vi "WSVCAP SHL Host TL I2C Read.vi"(0 "Bytes to Read":u8=8, 5 "Sub Address [U8]":u8=191 format="%.0x", 7 "Socket Mask Set [U64]":u64[](array[numeric]) format="%012x", 11 "error in":errorcluster, 13 "Log (T)":bool=TRUE) -> (4 "C1 Read Data Out":u8[][](array[numeric]) format="%.0x", 6 "C2 Read Data Out":u8[][](array[numeric]) format="%.0x", 8 "C3 Read Data Out":u8[][](array[numeric]) format="%.0x", 15 "error out":errorcluster)   [LabVIEW 2012]
uses:
  Type Defs/WSVCAP SHL Function Enum.ctl
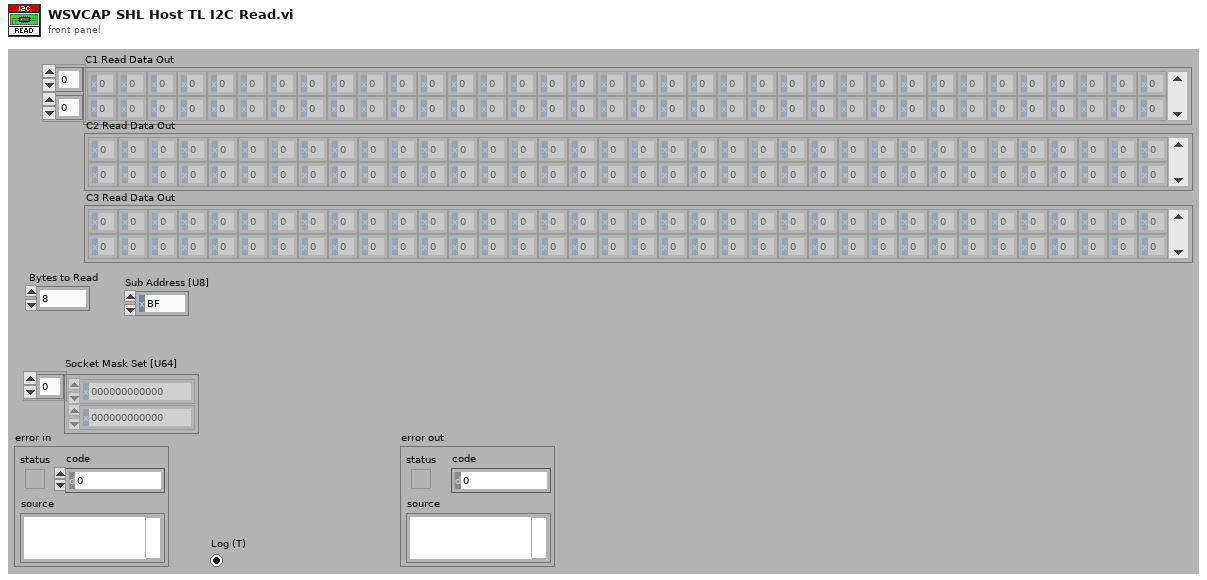
[diagram p1: front panel]
types:
  T1 = typedef "WSVCAP SHL Function Enum.ctl" = enum16{"Initialize", "Configure I2C", "Configure SPI", "Configure RFFE", "Write I2C", "Read I2C", "Write/Read SPI", "Start SPI Cycle", "Stop SPI Cycle", "Write RFFE", "Read RFFE", "Start RFFE Cycle", "Stop RFFE Cycle", "Get Status", "Close"}
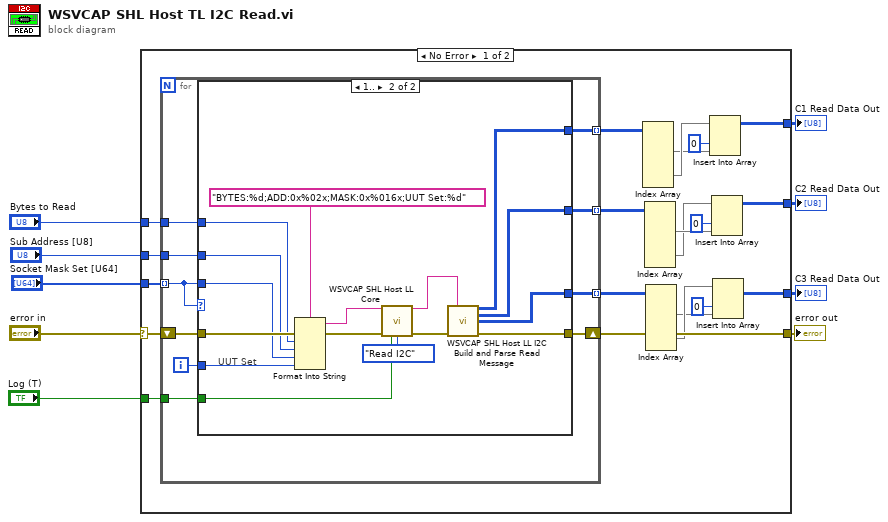
[diagram p0: block diagram]
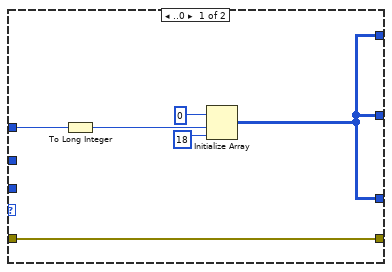
[diagram p2: hidden frame]
diagram:
  n1 = case shown="No Error" "error in" {
    selector: "error in" -> [w29 w63]
    tunnel: [w30 w63] -> w8
    tunnel: [w21 _] -> w3
    tunnel: [w12 _] -> w2
    tunnel: "Bytes to Read" -> [w28 _]
    tunnel: "Sub Address [U8]" -> [w27 _]
    tunnel: "Socket Mask Set [U64]" -> [w26 _]
    tunnel: "Log (T)" -> [w25 _]
    tunnel: [w10 _] -> w1
    frame No Error {
      n2 = for {
        tunnel: [w39] -> w13 mode=indexing
        tunnel: w28 -> [w37]
        tunnel: w27 -> [w36]
        tunnel: w26 -> [w33] mode=indexing
        tunnel: w25 -> [w35]
        tunnel: [w34] -> w11 mode=indexing
        tunnel: [w32] -> w20 mode=indexing
        shift-right: [w40] -> w30
        shift-left: w29 -> [w38]
        i -> [w31]
        n3 = case shown="1.." w33 {
          tunnel: [w46 w61] -> w40
          tunnel: [w42 w59] -> w32
          tunnel: [w42 w58] -> w39
          tunnel: w38 -> [w46 w57]
          tunnel: w37 -> [w43 w54]
          tunnel: w36 -> [_ w53]
          tunnel: w33 -> [_ w52]
          tunnel: w35 -> [_ w49]
          tunnel: [w42 w48] -> w34
          tunnel: w31 -> [_ w47]
          frame ..0 {
            n4 = To Long Integer(number=w43) -> (32bit integer=w41:i32)
            n5 = Initialize Array(u8 0 ("Read Data"), w41, 18 ("Read Data")) -> (w42:u8[][])
          }
          frame 1.. {
            # "UUT Set"
            n6 = Format Into String(format string="BYTES:%d;ADD:0x%02x;MASK:0x%016x;UUT Set:%d", error in=w57, w54, w53, w52, w47) -> (resulting string=w51:string, error out=w56:errorcluster)  [unwired: 1 in]
            n7 = call "WSVCAP SHL Host LL Core.vi"("Message In"=w51, "error in"=w56, "Log (T)"=w49, "Function"=WSVCAP_SHL_Function_Enum."Read I2C") -> ("Message Out"=w60:string, "error out"=w62:errorcluster)  [unwired: 9 in, 1 out]
            n8 = call "WSVCAP SHL Host LL I2C Build and Parse Read Message.vi"("Message In"=w60, "error in"=w62) -> ("C1 Read Data Out"=w59:u8[][], "C2 Read Data Out"=w58:u8[][], "C3 Read Data Out"=w48:u8[][], "error out"=w61:errorcluster)  [unwired: 8 in, 2 out]
          }
        }
      }
      n9 = Index Array(array=w20) -> (element #1=w23:u8[][], element #2=w24:u8[][])  [unwired: 6 in]
      n10 = Index Array(array=w13) -> (element #1=w18:u8[][], element #2=w17:u8[][])  [unwired: 6 in]
      n11 = Index Array(array=w11) -> (element #1=w15:u8[][], element #2=w16:u8[][])  [unwired: 6 in]
      n12 = Insert Into Array(array=w24, index (col)=0 ("disabled index (col)"), new element=w23) -> (w21:u8[][])  [unwired: 1 in]
      n13 = Insert Into Array(array=w17, index (col)=0 ("disabled index (col)"), new element=w18) -> (w12:u8[][])  [unwired: 1 in]
      n14 = Insert Into Array(array=w16, index (col)=0 ("disabled index (col)"), new element=w15) -> (w10:u8[][])  [unwired: 1 in]
    }
    frame Error {
    }
  }
  "error out" <- w8
  "C3 Read Data Out" <- w1
  "C1 Read Data Out" <- w3
  "C2 Read Data Out" <- w2
